vi "7_1_sub_children.vi"(10 "Child Paths Set 2":set{string}(c389), 11 "Tree Map Out":T1) -> (1 "Data":string, 2 "Child Paths Set":set{string}(c389), 3 "Tree Map Out 2":T1)   [LabVIEW 2025, in "2022.lvlib"]
uses:
  2022.lvlib
  <vilib>/National Instruments/Tree Map/Tree Map Data.ctl
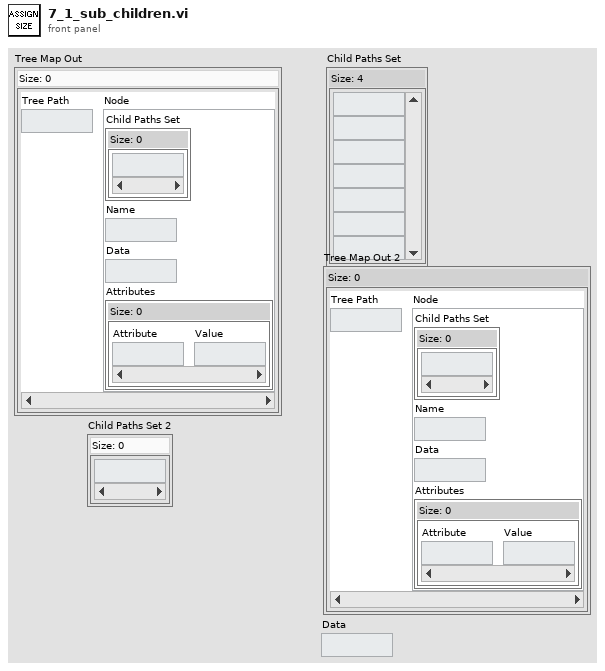
[diagram p1: front panel]
types:
  T1 = typedef "Tree Map.lvlib/Tree Map Data.ctl" = map{string, cluster{"Child Paths Set":set{string}, "Name":string, "Data":string, "Attributes":map{string, string}}}
  T2 = cluster{"Child Paths Set":set{string}, "Name":string, "Data":string, "Attributes":map{string, string}}
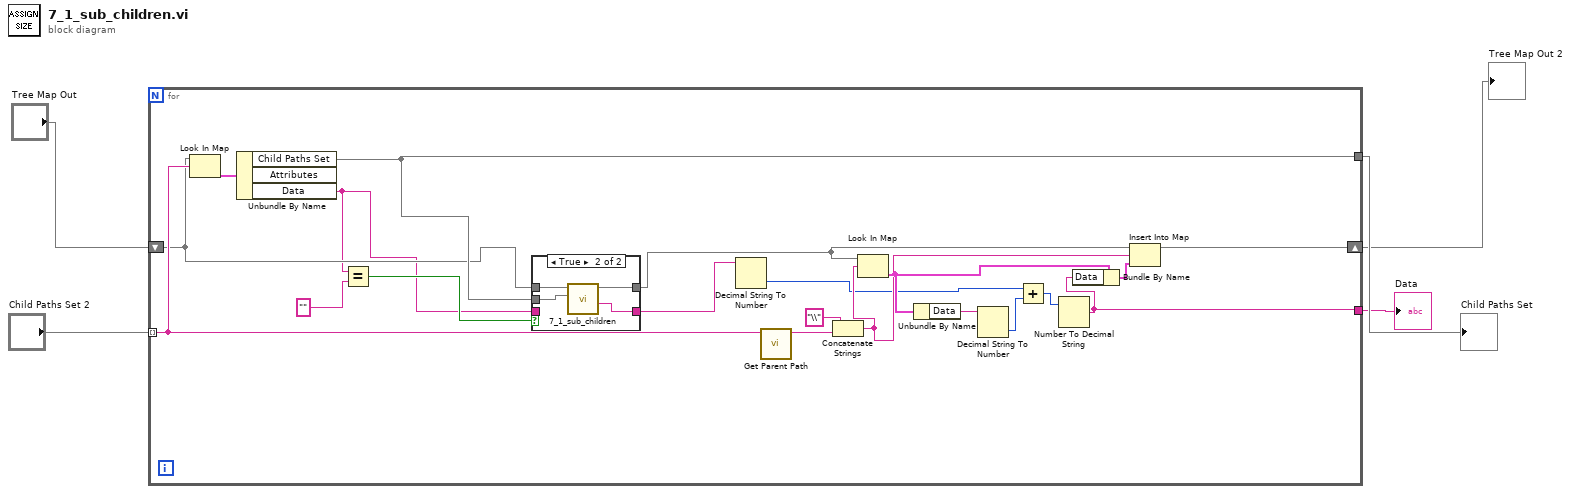
[diagram p0: block diagram]
diagram:
  n1 = for {
    tunnel: [w11] -> w3
    tunnel: "Child Paths Set 2" -> [w23] mode=indexing
    shift-right: [w22] -> w2
    shift-left: "Tree Map Out" -> [w10]
    tunnel: [w6] -> w1
    n2 = Look In Map(map=w10, key=w23) -> (value=w25:T2)  [unwired: 1 in, 1 out]
    n3 = Unbundle By Name(w25) -> ("Child Paths Set"=w11:set{string}, "Data"=w8:string)  [unwired: 1 out]
    n4 = Equal?(x=w8, y="") -> (x = y?=w12:bool)
    n5 = case shown="True" w12 {
      tunnel: w11 -> [_ w31]
      tunnel: w10 -> [w27 w30]
      tunnel: [w27 w29] -> w9
      tunnel: w8 -> [w26 _]
      tunnel: [w26 w28] -> w7
      frame False {
      }
      frame True {
        n6 = call "7_1_sub_children.vi"("Child Paths Set 2"=w31, "Tree Map Out"=w30) -> ("Data"=w28:string, "Tree Map Out 2"=w29:T1)  [unwired: 7 in, 1 out]
      }
    }
    n7 = Decimal String To Number(string=w7) -> (number=w14:i32)  [unwired: 2 in, 1 out]
    n8 = call <vilib>:"Get Parent Path.vi"("Node Path"=w23) -> ("Parent Path"=w17:string)  [unwired: 8 in, 2 out]
    n9 = Concatenate Strings("\\" ("string"), w17) -> (w16:string)
    n10 = Look In Map(map=w9, key=w16) -> (value=w20:T2)  [unwired: 1 in, 1 out]
    n11 = Unbundle By Name(w20) -> ("Data"=w21:string)
    n12 = Decimal String To Number(string=w21) -> (number=w13:i32)  [unwired: 2 in, 1 out]
    n13 = Add(x=w14, y=w13) -> (x+y=w19:i32)
    n14 = Number To Decimal String(number=w19) -> (decimal integer string=w6:string)  [unwired: 1 in]
    n15 = Bundle By Name(cluster=w20, "Data"=w6) -> (w18:T2)
    n16 = Insert Into Map(map in=w9, key=w16, value=w18) -> (map out=w22:T1)  [unwired: 2 out]
  }
  "Child Paths Set" <- w3
  "Tree Map Out 2" <- w2
  "Data" <- w1
